vi "PH_SHS_Analysis_Calibrator.ProcEvents.vi"(0 "i ref in":refnum<vi>, 5 "error in":errorcluster) -> (14 "i ref out":refnum<vi>, 19 "error out":errorcluster)   [LabVIEW 2014, in "PH_SHS_Analysis_Calibrator.lvlib"]
doc: "This method is used to define the events the object will listen to. Add your own events here."
uses:
  PH_SHS_Analysis_Calibrator.lvlib
  CSCore/BaseProcess/BaseProcess.event definition.ctl
  CSCore/CAEObj/CAEObj.event definition.ctl
  CSCore/BaseProcess/BaseProcess.descriptor string definition.ctl
  CSCore/BaseProcess/BaseProcess.lvlib
  CSCore/CAEObj/CAEObj.lvlib
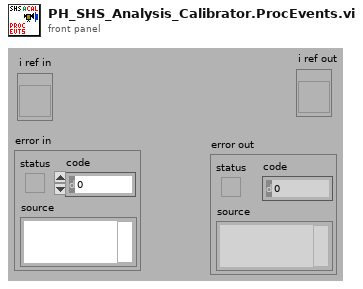
[diagram p1: front panel]
types:
  T1 = typedef "BaseProcess.lvlib/BaseProcess.event definition.ctl" = cluster{"CAEEvtDef":T2, "Data Descriptor":T3}
  T2 = typedef "CAEObj.lvlib/CAEObj.event definition.ctl" = cluster{"URL":string, "enable":bool, "ignoreResID":bool}
  T3 = typedef "BaseProcess.lvlib/BaseProcess.descriptor string definition.ctl" = string
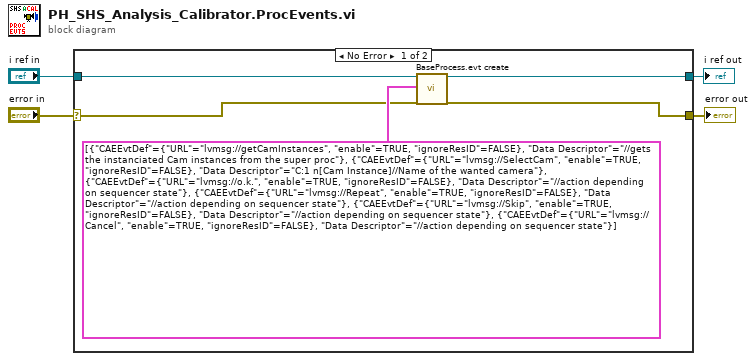
[diagram p0: block diagram]
diagram:
  n1 = case shown="No Error" "error in" {
    selector: "error in" -> [w5 w10]
    tunnel: "i ref in" -> [w9 w11]
    tunnel: [w8 w11] -> w3
    tunnel: [w7 w10] -> w2
    frame No Error {
      n2 = call "BaseProcess.evt create.vi"("i ref in"=w9, "newEvents"=T1[] [{"CAEEvtDef"={"URL"="lvmsg://getCamInstances", "enable"=TRUE, "ignoreResID"=FALSE}, "Data Descriptor"="//gets the instanciated Cam instances from the super proc"}, {"CAEEvtDef"={"URL"="lvmsg://SelectCam", "enable"=TRUE, "ignoreResID"=FALSE}, "Data Descriptor"="C:1 n[Cam Instance]//Name of the wanted camera"}, {"CAEEvtDef"={"URL"="lvmsg://o.k.", "enable"=TRUE, "ignoreResID"=FALSE}, "Data Descriptor"="//action depending on sequencer state"}, {"CAEEvtDef"={"URL"="lvmsg://Repeat", "enable"=TRUE, "ignoreResID"=FALSE}, "Data Descriptor"="//action depending on sequencer state"}, {"CAEEvtDef"={"URL"="lvmsg://Skip", "enable"=TRUE, "ignoreResID"=FALSE}, "Data Descriptor"="//action depending on sequencer state"}, {"CAEEvtDef"={"URL"="lvmsg://Cancel", "enable"=TRUE, "ignoreResID"=FALSE}, "Data Descriptor"="//action depending on sequencer state"}] ("new events(V3.0)"), "error in (no error)"=w5) -> ("i ref out"=w8:refnum<vi>, "error out"=w7:errorcluster)  [unwired: 13 in, 2 out]
    }
    frame Error {
    }
  }
  "i ref out" <- w3
  "error out" <- w2
